vi "DeltaE(CMC).vi"(1 "l:c":bool, 2 "L*a*b colors":T1) -> (0 "Delta E":dbl)   [LabVIEW 2013]
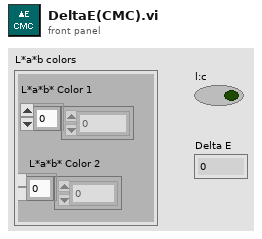
[diagram p1: front panel]
types:
  T1 = cluster{"L*a*b* Color 1":dbl[], "L*a*b* Color 2":dbl[]}
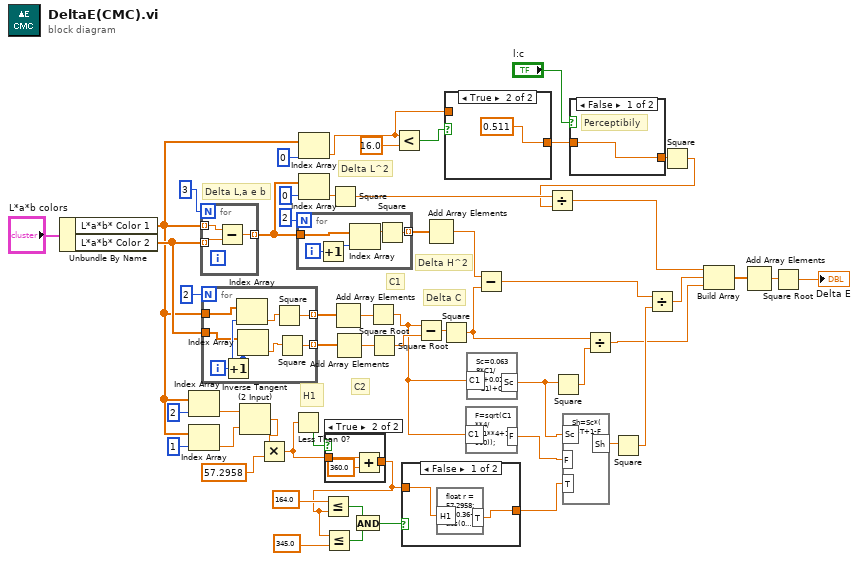
[diagram p0: block diagram]
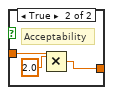
[diagram p2: hidden frame]
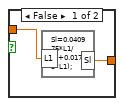
[diagram p3: hidden frame]
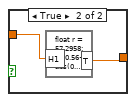
[diagram p5: hidden frame]
diagram:
  # "Delta L^2"
  # "H1"
  # "Delta H^2"
  # "Delta C"
  # "C2"
  # "C1"
  # "Delta L,a e b"
  n1 = Unbundle By Name("L*a*b colors") -> ("L*a*b* Color 1"=w27:dbl[], "L*a*b* Color 2"=w52:dbl[])
  n2 = Index Array(array=w27, index=2) -> (element=w1:dbl)
  n3 = Index Array(array=w27, index=1) -> (element=w2:dbl)
  n4 = for {
    N: 3 -> [_]
    tunnel: w27 -> [w58] mode=indexing
    tunnel: w52 -> [w57] mode=indexing
    tunnel: [w56] -> w42 mode=indexing
    n5 = Subtract(x=w58, y=w57) -> (x-y=w56:dbl)
  }
  n6 = for {
    N: 2 -> [_]
    tunnel: w27 -> [w65]
    tunnel: w52 -> [w63]
    tunnel: [w60] -> w51 mode=indexing
    tunnel: [w59] -> w50 mode=indexing
    i -> [w66]
    n7 = Increment(x=w66) -> (x+1=w64:i32)
    n8 = Index Array(array=w65, index=w64) -> (element=w62:dbl)
    n9 = Index Array(array=w63, index=w64) -> (element=w61:dbl)
    n10 = Square(x=w62) -> (x^2=w60:dbl)
    n11 = Square(x=w61) -> (x^2=w59:dbl)
  }
  n12 = Inverse Tangent (2 Input)(1:w2, 2:w1) -> (0:w5:dbl)
  n13 = Multiply(x=w5, y=57.2958) -> (x*y=w3:dbl)
  n14 = Less Than 0?(x=w3) -> (x < 0?=w32:bool)
  n15 = for {
    N: 2 -> [_]
    tunnel: w42 -> [w70]
    tunnel: [w67] -> w45 mode=indexing
    i -> [w71]
    n16 = Increment(x=w71) -> (x+1=w69:i32)
    n17 = Index Array(array=w70, index=w69) -> (element=w68:dbl)
    n18 = Square(x=w68) -> (x^2=w67:dbl)
  }
  n19 = Index Array(array=w27, index=0) -> (element=w23:dbl)
  n20 = Index Array(array=w42, index=0) -> (element=w40:dbl)
  n21 = case shown="True" w32 {
    tunnel: w3 -> [w72 w75]
    tunnel: [w72 w73] -> w31
    frame False {
    }
    frame True {
      n22 = Add(x=w75, y=360.0) -> (x+y=w73:dbl)
    }
  }
  n23 = Less Or Equal?(x=164.0, y=w31) -> (x <= y?=w34:bool)
  n24 = Less Or Equal?(x=w31, y=345.0 ("x")) -> (x <= y?=w35:bool)
  n25 = Square(x=w40) -> (x^2=w17:dbl)
  n26 = Add Array Elements(numeric array=w51) -> (sum=w49:dbl)
  n27 = Add Array Elements(numeric array=w50) -> (sum=w48:dbl)
  n28 = And(x=w34, y=w35) -> (x .and. y?=w33:bool)
  n29 = Square Root(x=w49) -> (sqrt(x)=w30:dbl)
  n30 = Square Root(x=w48) -> (sqrt(x)=w47:dbl)
  n31 = Less?(x=w23, y=16.0) -> (x < y?=w24:bool)
  n32 = case shown="False" w33 {
    tunnel: w31 -> [w77 w79]
    tunnel: [w76 w78] -> w28
    frame False {
      n33 = formula code="float r = 57.2958;\nT=0.36+abs(0.4*cos((H1+35)/r));"("H1"=w77) -> ("T"=w76:dbl)
    }
    frame True {
      n34 = formula code="float r = 57.2958;\nT=0.56+abs(0.2*cos((H1+168)/r));"("H1"=w79) -> ("T"=w78:dbl)
    }
  }
  n35 = Subtract(x=w30, y=w47) -> (x-y=w44:dbl)
  n36 = Add Array Elements(numeric array=w45) -> (sum=w43:dbl)
  n37 = Square(x=w44) -> (x^2=w14:dbl)
  n38 = case shown="True" w24 {
    tunnel: [w80 0.511] -> w21
    tunnel: w23 -> [w81 _]
    frame False {
      n39 = formula code="Sl=0.040975*L1/(1+0.01765*L1);"("L1"=w81) -> ("Sl"=w80:dbl)
    }
    frame True {
    }
  }
  n40 = formula code="F=sqrt(C1**4/(C1**4+1900));"("C1"=w30) -> ("F"=w29:dbl)
  n41 = formula code="Sc=0.0638*C1/(1+0.0131*C1)+0.638;"("C1"=w30) -> ("Sc"=w18:dbl)
  n42 = Subtract(x=w43, y=w14) -> (x-y=w12:dbl)
  n43 = Square(x=w18) -> (x^2=w15:dbl)
  n44 = formula code="Sh=Sc*(F*T+1-F);"("Sc"=w18, "F"=w29, "T"=w28) -> ("Sh"=w19:dbl)
  n45 = case shown="False" "l:c" {
    tunnel: w21 -> [w83 w86]
    tunnel: [w83 w84] -> w20
    frame False {
      # "Perceptibily"
    }
    frame True {
      # "Acceptability"
      n46 = Multiply(x=2.0, y=w86) -> (x*y=w84:dbl)
    }
  }
  n47 = Divide(x=w14, y=w15) -> (x/y=w9:dbl)
  n48 = Square(x=w19) -> (x^2=w13:dbl)
  n49 = Divide(x=w12, y=w13) -> (x/y=w10:dbl)
  n50 = Square(x=w20) -> (x^2=w16:dbl)
  n51 = Divide(x=w17, y=w16) -> (x/y=w11:dbl)
  n52 = Build Array(w11, w10, w9) -> (w8:dbl[])
  n53 = Add Array Elements(numeric array=w8) -> (sum=w7:dbl)
  n54 = Square Root(x=w7) -> (sqrt(x)=→"Delta E":dbl)
